vi "CheckCameraIndexValid.vi"(8 "Camera Manager Data":T2={"Camera Index"=0.0, "Exposure Time"=2800.0, "Image"=refnum, "Save Img Path"=path "C:/Users/MyUser/Pictures", "error out"={"status"=FALSE, "code"=0, "source"=""}, "Specific Parameter"={"Parameter Name"="", "Parameter Value"=""}, "Image Info"={"Height"=0.0, "Width"=0.0, "Channels"=0.0}}, 11 "CameraCount":dbl) -> (0 "Camera Manager Data Out":T2={"Camera Index"=0.0, "Exposure Time"=2800.0, "Image"=refnum, "Save Img Path"=path "C:/Users/MyUser/Pictures", "error out"={"status"=FALSE, "code"=0, "source"=""}, "Specific Parameter"={"Parameter Name"="", "Parameter Value"=""}, "Image Info"={"Height"=0.0, "Width"=0.0, "Channels"=0.0}}, 2 "IsValidIndex":bool)   [LabVIEW 2017, in "PlayNitrideCameraComponet1010_4.lvlib"]
uses:
  <userlib>/PlayNitrideCameraComponet1010_4/PlayNitrideCameraComponet1010_4.lvlib
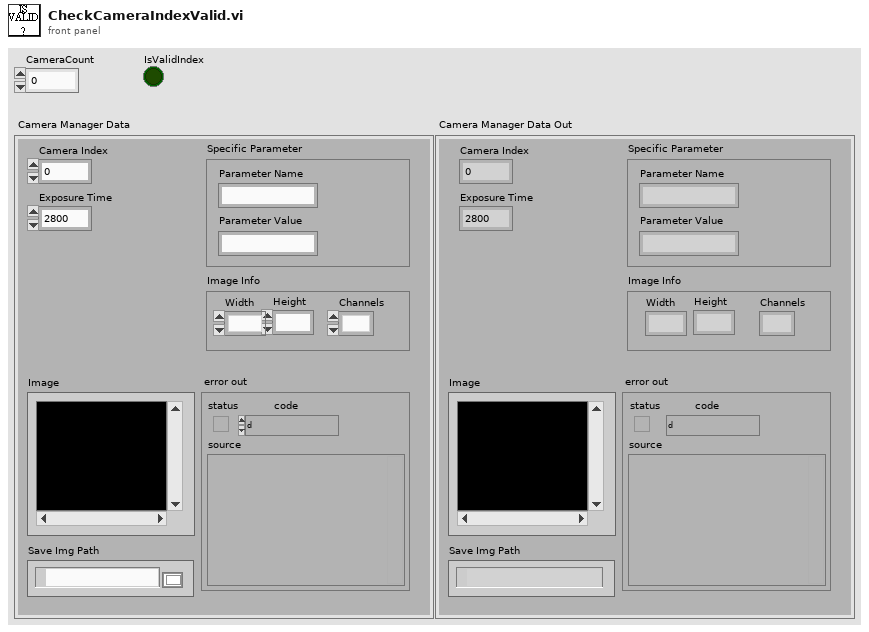
[diagram p1: front panel]
types:
  T1 = typedef "IMAQ Image.ctl" = refnum<image>
  T2 = cluster{"Camera Index":dbl, "Exposure Time":dbl, "Image":T1, "Save Img Path":path, "error out":errorcluster, "Specific Parameter":cluster{"Parameter Name":string, "Parameter Value":string}, "Image Info":cluster{"Height":dbl, "Width":dbl, "Channels":dbl}}
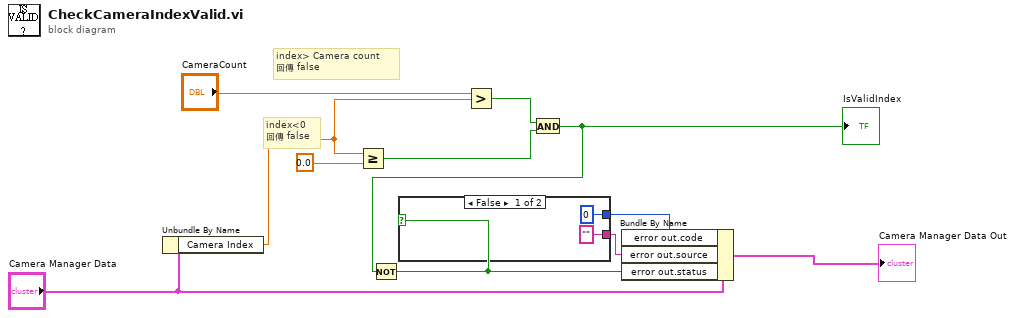
[diagram p0: block diagram]
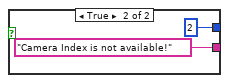
[diagram p2: hidden frame]
diagram:
  # "index> Camera count\n回傳 false"
  # "index<0\n回傳 false"
  n1 = Unbundle By Name("Camera Manager Data") -> ("Camera Index"=w3:dbl)
  n2 = Greater Or Equal?(x=w3, y=0.0) -> (x >= y?=w5:bool)
  n3 = Greater?(x="CameraCount", y=w3) -> (0:w6:bool)
  n4 = And(x=w6, y=w5) -> (x .and. y?=w2:bool)
  "IsValidIndex" <- w2
  n5 = Not(x=w2) -> (.not. x?=w10:bool)
  n6 = case shown="False" w10 {
    tunnel: ["" ("error out.source") "Camera Index is not available!" ("error out.source")] -> w9
    tunnel: [0 2] -> w1
    frame False {
    }
    frame True {
    }
  }
  n7 = Bundle By Name(cluster="Camera Manager Data", "error out.code"=w1, "error out.source"=w9, "error out.status"=w10) -> (→"Camera Manager Data Out":T2)
